vi "read_IMU Main_simple.vi"() -> ()   [LabVIEW 2013]
uses:
  IMU_Data_Type_Def.ctl
  <vilib>/myRIO/Common/Instrument Driver Framework/myRIO v1.0/UART/vis/myRIO v1.0 Close UART.vi
  <vilib>/myRIO/Common/Instrument Driver Framework/Utilities/vis/FPGA Ref Manager.vi
  <vilib>/myRIO/Common/Instrument Driver Framework/myRIO v1.0/myRIO v1.0 Reset FPGA.vi
  <vilib>/myRIO/Instrument Drivers/Utilities/Utilities.lvlib
panel:
  in  "Gravitation-Constant":dbl=9.81
  out "Less then 90Hz":bool
  out "Less then 100Hz":bool
  out "IMU_Data_simple":T1
  out "Elapsed Loop time [ms]":u32
  out "error out":errorcluster
  in  "stop":bool
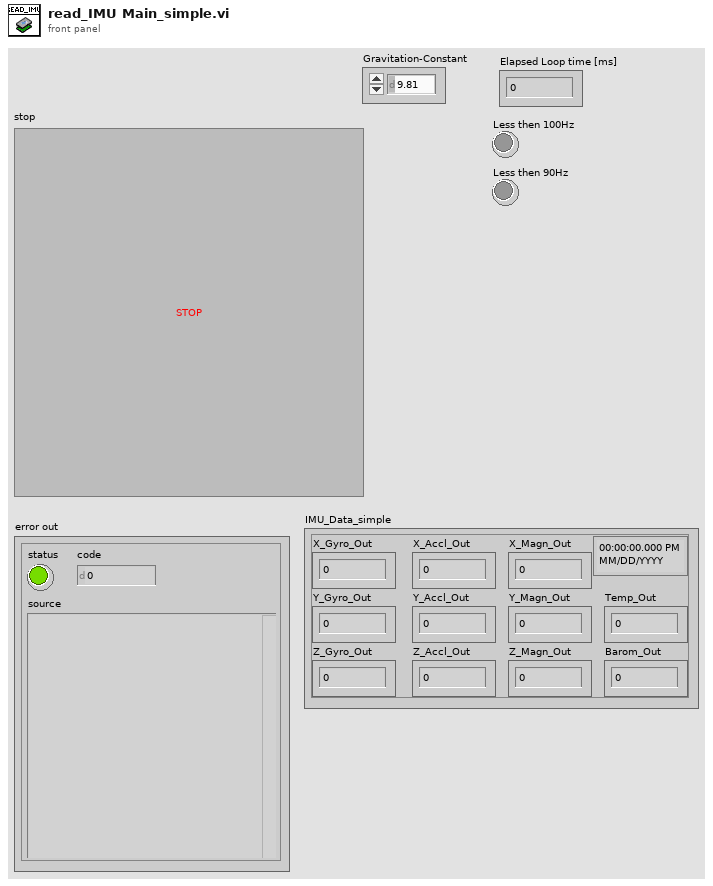
[diagram p1: front panel]
types:
  T1 = typedef "IMU_Data_Type_Def.ctl" = cluster{timestamp, "X_Gyro_Out":dbl, "Y_Gyro_Out":dbl, "Z_Gyro_Out":dbl, "X_Accl_Out":dbl, "Y_Accl_Out":dbl, "Z_Accl_Out":dbl, "X_Magn_Out":dbl, "Y_Magn_Out":dbl, "Z_Magn_Out":dbl, "Temp_Out":dbl, "Barom_Out":dbl}
  T2 = cluster{timestamp, "Scaled Measurement 1":dbl, "Scaled last Measurement":dbl, "Scaled Measurement 1":dbl, "Scaled last Measurement":dbl, "Scaled Measurement 1":dbl, "Scaled last Measurement":dbl, "Scaled Measurement 1":dbl, "Scaled last Measurement":dbl, "Scaled Measurement 1":dbl, "Scaled last Measurement":dbl, "Scaled Measurement 1":dbl}
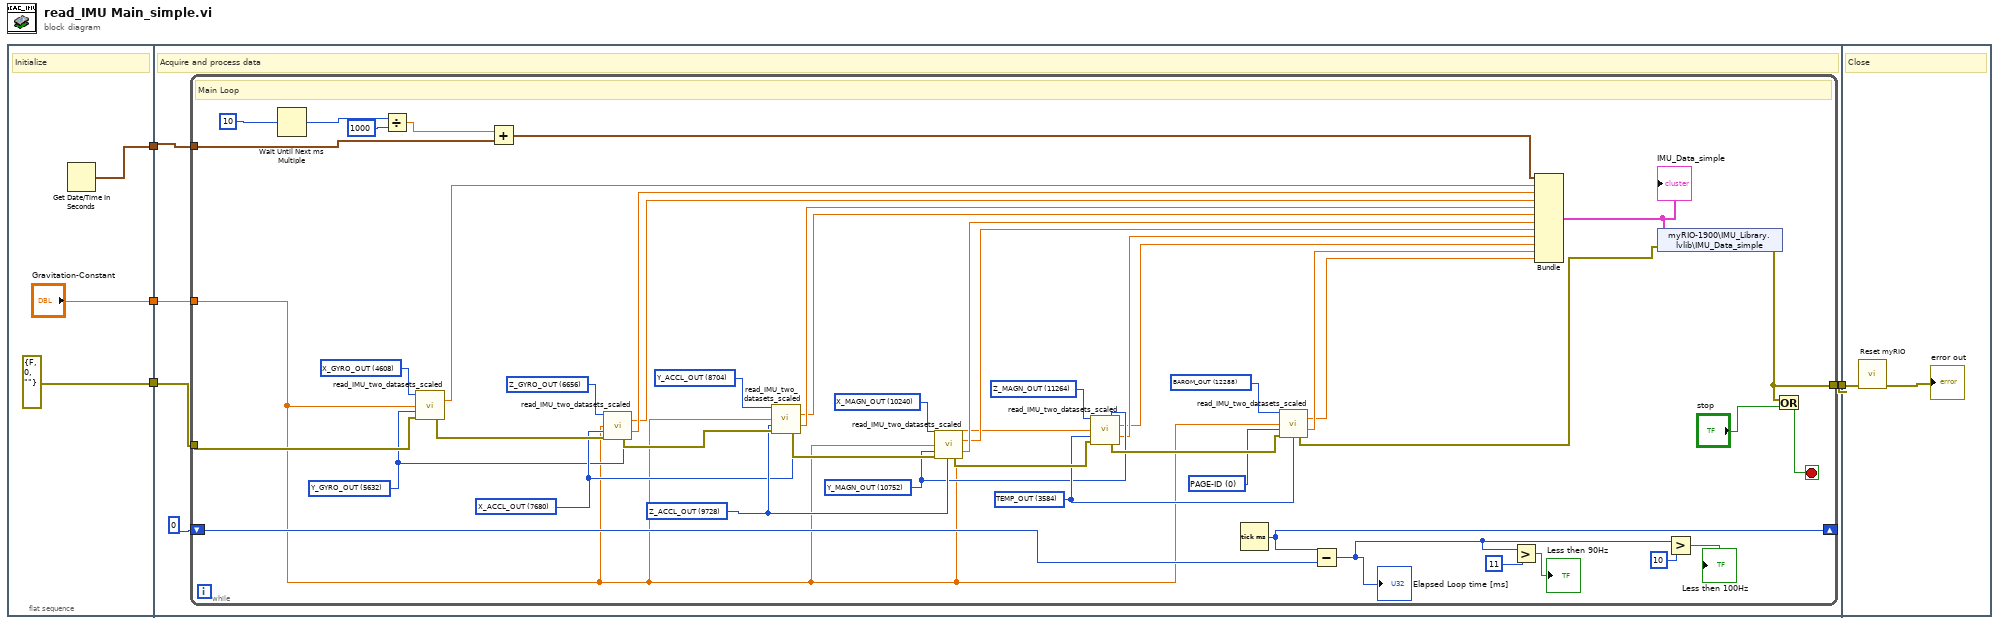
[diagram p0: block diagram]
diagram:
  n1 = flat-sequence {
    tunnel: [errorcluster {"status"=FALSE, "code"=0, "source"=""} ("error out")] -> w4
    tunnel: [w6] -> w3
    tunnel: ["Gravitation-Constant"] -> w1
    tunnel: w4 -> [w12]
    tunnel: w3 -> [w10]
    tunnel: [w9] -> w2
    tunnel: w1 -> [w8]
    tunnel: w2 -> [w61]
    frame #0 {
      # "Initialize"
      n2 = Get Date/Time In Seconds() -> (seconds since 1Jan1904=w6:timestamp)
    }
    frame #1 {
      # "Acquire and process data"
      n3 = while {
        tunnel: w12 -> [w59]
        shift-right: [w44] -> _
        shift-left: u32 0 ("millisecond timer value") -> [w45]
        tunnel: w10 -> [w42]
        tunnel: [w20] -> w9
        tunnel: w8 -> [w13]
        stop <- w47 stop-if-true
        w41 = u16 0 items=["PAGE-ID"=0, "SYS_E_FLAG"=2048, "DIAG_STS"=2560, "ALM_STS"=3072, "TEMP_OUT"=3584, "X_GYRO_OUT"=4608, "Y_GYRO_OUT"=5632, "Z_GYRO_OUT"=6656, "X_ACCL_OUT"=7680, "Y_ACCL_OUT"=8704, "Z_ACCL_OUT"=9728, "X_MAGN_OUT"=10240, "Y_MAGN_OUT"=10752, "Z_MAGN_OUT"=11264, "BAROM_OUT"=12288, "X_DELTAANG_OUT"=16896, "Y_DELTAANG_OUT"=17920, "Z_DELTAANG_OUT"=18944, "X_DELTAVEL_OUT"=19968, "Y_DELTAVEL_OUT"=20992, "Z_DELTAVEL_OUT"=22016] ("Measurement Type 1")
        w53 = u16 12288 items=["PAGE-ID"=0, "SYS_E_FLAG"=2048, "DIAG_STS"=2560, "ALM_STS"=3072, "TEMP_OUT"=3584, "X_GYRO_OUT"=4608, "Y_GYRO_OUT"=5632, "Z_GYRO_OUT"=6656, "X_ACCL_OUT"=7680, "Y_ACCL_OUT"=8704, "Z_ACCL_OUT"=9728, "X_MAGN_OUT"=10240, "Y_MAGN_OUT"=10752, "Z_MAGN_OUT"=11264, "BAROM_OUT"=12288, "X_DELTAANG_OUT"=16896, "Y_DELTAANG_OUT"=17920, "Z_DELTAANG_OUT"=18944, "X_DELTAVEL_OUT"=19968, "Y_DELTAVEL_OUT"=20992, "Z_DELTAVEL_OUT"=22016] ("Measurement Type 1")
        w43 = u16 3584 items=["PAGE-ID"=0, "SYS_E_FLAG"=2048, "DIAG_STS"=2560, "ALM_STS"=3072, "TEMP_OUT"=3584, "X_GYRO_OUT"=4608, "Y_GYRO_OUT"=5632, "Z_GYRO_OUT"=6656, "X_ACCL_OUT"=7680, "Y_ACCL_OUT"=8704, "Z_ACCL_OUT"=9728, "X_MAGN_OUT"=10240, "Y_MAGN_OUT"=10752, "Z_MAGN_OUT"=11264, "BAROM_OUT"=12288, "X_DELTAANG_OUT"=16896, "Y_DELTAANG_OUT"=17920, "Z_DELTAANG_OUT"=18944, "X_DELTAVEL_OUT"=19968, "Y_DELTAVEL_OUT"=20992, "Z_DELTAVEL_OUT"=22016] ("Measurement Type 2")
        w54 = u16 11264 items=["PAGE-ID"=0, "SYS_E_FLAG"=2048, "DIAG_STS"=2560, "ALM_STS"=3072, "TEMP_OUT"=3584, "X_GYRO_OUT"=4608, "Y_GYRO_OUT"=5632, "Z_GYRO_OUT"=6656, "X_ACCL_OUT"=7680, "Y_ACCL_OUT"=8704, "Z_ACCL_OUT"=9728, "X_MAGN_OUT"=10240, "Y_MAGN_OUT"=10752, "Z_MAGN_OUT"=11264, "BAROM_OUT"=12288, "X_DELTAANG_OUT"=16896, "Y_DELTAANG_OUT"=17920, "Z_DELTAANG_OUT"=18944, "X_DELTAVEL_OUT"=19968, "Y_DELTAVEL_OUT"=20992, "Z_DELTAVEL_OUT"=22016] ("Measurement Type 1")
        w37 = u16 10752 items=["PAGE-ID"=0, "SYS_E_FLAG"=2048, "DIAG_STS"=2560, "ALM_STS"=3072, "TEMP_OUT"=3584, "X_GYRO_OUT"=4608, "Y_GYRO_OUT"=5632, "Z_GYRO_OUT"=6656, "X_ACCL_OUT"=7680, "Y_ACCL_OUT"=8704, "Z_ACCL_OUT"=9728, "X_MAGN_OUT"=10240, "Y_MAGN_OUT"=10752, "Z_MAGN_OUT"=11264, "BAROM_OUT"=12288, "X_DELTAANG_OUT"=16896, "Y_DELTAANG_OUT"=17920, "Z_DELTAANG_OUT"=18944, "X_DELTAVEL_OUT"=19968, "Y_DELTAVEL_OUT"=20992, "Z_DELTAVEL_OUT"=22016] ("Measurement Type 2")
        w55 = u16 10240 items=["PAGE-ID"=0, "SYS_E_FLAG"=2048, "DIAG_STS"=2560, "ALM_STS"=3072, "TEMP_OUT"=3584, "X_GYRO_OUT"=4608, "Y_GYRO_OUT"=5632, "Z_GYRO_OUT"=6656, "X_ACCL_OUT"=7680, "Y_ACCL_OUT"=8704, "Z_ACCL_OUT"=9728, "X_MAGN_OUT"=10240, "Y_MAGN_OUT"=10752, "Z_MAGN_OUT"=11264, "BAROM_OUT"=12288, "X_DELTAANG_OUT"=16896, "Y_DELTAANG_OUT"=17920, "Z_DELTAANG_OUT"=18944, "X_DELTAVEL_OUT"=19968, "Y_DELTAVEL_OUT"=20992, "Z_DELTAVEL_OUT"=22016] ("Measurement Type 1")
        w40 = u16 9728 items=["PAGE-ID"=0, "SYS_E_FLAG"=2048, "DIAG_STS"=2560, "ALM_STS"=3072, "TEMP_OUT"=3584, "X_GYRO_OUT"=4608, "Y_GYRO_OUT"=5632, "Z_GYRO_OUT"=6656, "X_ACCL_OUT"=7680, "Y_ACCL_OUT"=8704, "Z_ACCL_OUT"=9728, "X_MAGN_OUT"=10240, "Y_MAGN_OUT"=10752, "Z_MAGN_OUT"=11264, "BAROM_OUT"=12288, "X_DELTAANG_OUT"=16896, "Y_DELTAANG_OUT"=17920, "Z_DELTAANG_OUT"=18944, "X_DELTAVEL_OUT"=19968, "Y_DELTAVEL_OUT"=20992, "Z_DELTAVEL_OUT"=22016] ("Measurement Type 2")
        w57 = u16 8704 items=["PAGE-ID"=0, "SYS_E_FLAG"=2048, "DIAG_STS"=2560, "ALM_STS"=3072, "TEMP_OUT"=3584, "X_GYRO_OUT"=4608, "Y_GYRO_OUT"=5632, "Z_GYRO_OUT"=6656, "X_ACCL_OUT"=7680, "Y_ACCL_OUT"=8704, "Z_ACCL_OUT"=9728, "X_MAGN_OUT"=10240, "Y_MAGN_OUT"=10752, "Z_MAGN_OUT"=11264, "BAROM_OUT"=12288, "X_DELTAANG_OUT"=16896, "Y_DELTAANG_OUT"=17920, "Z_DELTAANG_OUT"=18944, "X_DELTAVEL_OUT"=19968, "Y_DELTAVEL_OUT"=20992, "Z_DELTAVEL_OUT"=22016] ("Measurement Type 1")
        w39 = u16 7680 items=["PAGE-ID"=0, "SYS_E_FLAG"=2048, "DIAG_STS"=2560, "ALM_STS"=3072, "TEMP_OUT"=3584, "X_GYRO_OUT"=4608, "Y_GYRO_OUT"=5632, "Z_GYRO_OUT"=6656, "X_ACCL_OUT"=7680, "Y_ACCL_OUT"=8704, "Z_ACCL_OUT"=9728, "X_MAGN_OUT"=10240, "Y_MAGN_OUT"=10752, "Z_MAGN_OUT"=11264, "BAROM_OUT"=12288, "X_DELTAANG_OUT"=16896, "Y_DELTAANG_OUT"=17920, "Z_DELTAANG_OUT"=18944, "X_DELTAVEL_OUT"=19968, "Y_DELTAVEL_OUT"=20992, "Z_DELTAVEL_OUT"=22016] ("Measurement Type 2")
        w58 = u16 6656 items=["PAGE-ID"=0, "SYS_E_FLAG"=2048, "DIAG_STS"=2560, "ALM_STS"=3072, "TEMP_OUT"=3584, "X_GYRO_OUT"=4608, "Y_GYRO_OUT"=5632, "Z_GYRO_OUT"=6656, "X_ACCL_OUT"=7680, "Y_ACCL_OUT"=8704, "Z_ACCL_OUT"=9728, "X_MAGN_OUT"=10240, "Y_MAGN_OUT"=10752, "Z_MAGN_OUT"=11264, "BAROM_OUT"=12288, "X_DELTAANG_OUT"=16896, "Y_DELTAANG_OUT"=17920, "Z_DELTAANG_OUT"=18944, "X_DELTAVEL_OUT"=19968, "Y_DELTAVEL_OUT"=20992, "Z_DELTAVEL_OUT"=22016] ("Measurement Type 1")
        w38 = u16 5632 items=["PAGE-ID"=0, "SYS_E_FLAG"=2048, "DIAG_STS"=2560, "ALM_STS"=3072, "TEMP_OUT"=3584, "X_GYRO_OUT"=4608, "Y_GYRO_OUT"=5632, "Z_GYRO_OUT"=6656, "X_ACCL_OUT"=7680, "Y_ACCL_OUT"=8704, "Z_ACCL_OUT"=9728, "X_MAGN_OUT"=10240, "Y_MAGN_OUT"=10752, "Z_MAGN_OUT"=11264, "BAROM_OUT"=12288, "X_DELTAANG_OUT"=16896, "Y_DELTAANG_OUT"=17920, "Z_DELTAANG_OUT"=18944, "X_DELTAVEL_OUT"=19968, "Y_DELTAVEL_OUT"=20992, "Z_DELTAVEL_OUT"=22016] ("Measurement Type 2")
        w49 = u16 4608 items=["PAGE-ID"=0, "SYS_E_FLAG"=2048, "DIAG_STS"=2560, "ALM_STS"=3072, "TEMP_OUT"=3584, "X_GYRO_OUT"=4608, "Y_GYRO_OUT"=5632, "Z_GYRO_OUT"=6656, "X_ACCL_OUT"=7680, "Y_ACCL_OUT"=8704, "Z_ACCL_OUT"=9728, "X_MAGN_OUT"=10240, "Y_MAGN_OUT"=10752, "Z_MAGN_OUT"=11264, "BAROM_OUT"=12288, "X_DELTAANG_OUT"=16896, "Y_DELTAANG_OUT"=17920, "Z_DELTAANG_OUT"=18944, "X_DELTAVEL_OUT"=19968, "Y_DELTAVEL_OUT"=20992, "Z_DELTAVEL_OUT"=22016] ("Measurement Type 1")
        # "Main Loop"
        n4 = Wait Until Next ms Multiple(millisecond multiple=u32 10 ("milliseconds to wait")) -> (millisecond timer value=w19:u32)
        n5 = Divide(x=w19, y=u32 1000) -> (x/y=w22:dbl)
        n6 = call "read_IMU_two_datasets_scaled.vi"("First Measurement Type"=w49, "Gravitation-Constant"=w13, "Next Measurement Type"=w38, "error in (no error)"=w59) -> ("Scaled Measurement 1"=w36:dbl, "error out"=w48:errorcluster)  [unwired: 5 in, 5 out]
        n7 = Add(x=w22, y=w42) -> (x+y=w25:timestamp)
        n8 = call "read_IMU_two_datasets_scaled.vi"("First Measurement Type"=w58, "Last Measurement Type"=w38, "Gravitation-Constant"=w13, "Next Measurement Type"=w39, "error in (no error)"=w48) -> ("Scaled Measurement 1"=w34:dbl, "Scaled last Measurement"=w35:dbl, "error out"=w56:errorcluster)  [unwired: 4 in, 4 out]
        n9 = call "read_IMU_two_datasets_scaled.vi"("First Measurement Type"=w57, "Last Measurement Type"=w39, "Gravitation-Constant"=w13, "Next Measurement Type"=w40, "error in (no error)"=w56) -> ("Scaled Measurement 1"=w32:dbl, "Scaled last Measurement"=w33:dbl, "error out"=w52:errorcluster)  [unwired: 4 in, 4 out]
        n10 = call "read_IMU_two_datasets_scaled.vi"("First Measurement Type"=w55, "Last Measurement Type"=w40, "Gravitation-Constant"=w13, "Next Measurement Type"=w37, "error in (no error)"=w52) -> ("Scaled Measurement 1"=w30:dbl, "Scaled last Measurement"=w31:dbl, "error out"=w51:errorcluster)  [unwired: 4 in, 4 out]
        n11 = call "read_IMU_two_datasets_scaled.vi"("First Measurement Type"=w54, "Last Measurement Type"=w37, "Gravitation-Constant"=w13, "Next Measurement Type"=w43, "error in (no error)"=w51) -> ("Scaled Measurement 1"=w28:dbl, "Scaled last Measurement"=w29:dbl, "error out"=w50:errorcluster)  [unwired: 4 in, 4 out]
        n12 = Tick Count (ms)() -> (millisecond timer value=w44:u32)
        n13 = call "read_IMU_two_datasets_scaled.vi"("First Measurement Type"=w53, "Last Measurement Type"=w43, "Gravitation-Constant"=w13, "Next Measurement Type"=w41, "error in (no error)"=w50) -> ("Scaled Measurement 1"=w26:dbl, "Scaled last Measurement"=w27:dbl, "error out"=w21:errorcluster)  [unwired: 4 in, 4 out]
        n14 = Subtract(x=w44, y=w45) -> (x-y=w16:u32)
        "Elapsed Loop time [ms]" <- w16
        n15 = Greater?(x=w16, y=u32 11) -> (0:→"Less then 90Hz":bool)
        n16 = Bundle(w25, "Scaled Measurement 1"=w36, "Scaled last Measurement"=w35, "Scaled Measurement 1"=w34, "Scaled last Measurement"=w33, "Scaled Measurement 1"=w32, "Scaled last Measurement"=w31, "Scaled Measurement 1"=w30, "Scaled last Measurement"=w29, "Scaled Measurement 1"=w28, "Scaled last Measurement"=w27, "Scaled Measurement 1"=w26) -> (w24:T2)  [unwired: 1 in]
        "IMU_Data_simple" <- w24
        n17 = shared-variable "myRIO-1900\\IMU_Library.lvlib\\IMU_Data_simple"(w24, error in=w21) -> (error out=w20:errorcluster)
        n18 = Greater?(x=w16, y=u32 10) -> (0:→"Less then 100Hz":bool)
        n19 = Or(x=w20, y="stop") -> (x .or. y?=w47:bool)
      }
    }
    frame #2 {
      # "Close"
      n20 = call <vilib>:"Reset myRIO.vi"("error in (no error)"=w61) -> ("error out"=→"error out":errorcluster)  [unwired: 10 in]
    }
  }
